vi "Connecting Points.vi"(1 "index":dbl[](array[numeric]), 2 "数组":dbl[][](array[numeric])) -> (0 "输出数组":T1(array[cluster]))   [LabVIEW 2016]
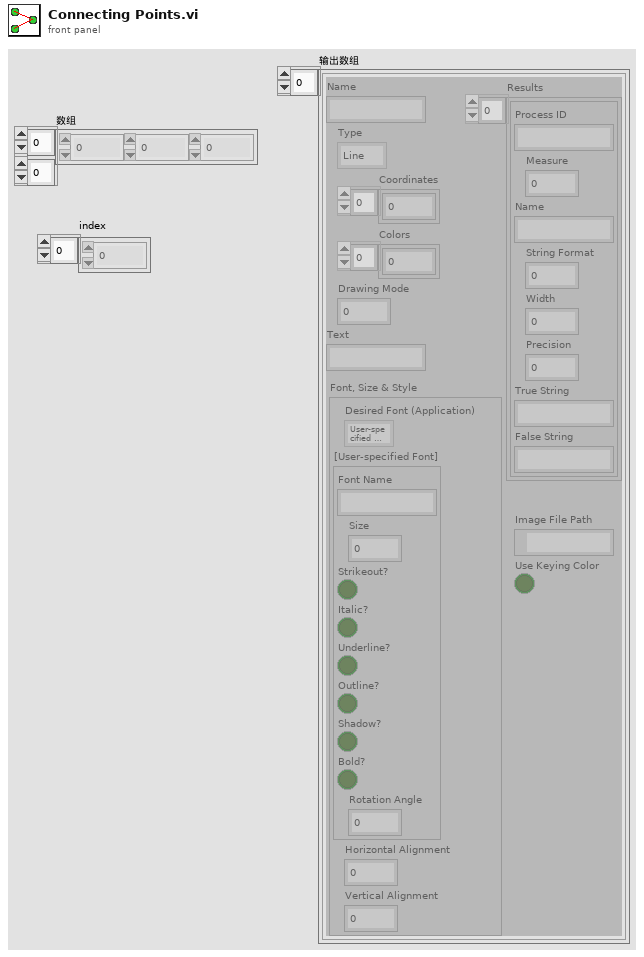
[diagram p1: front panel]
types:
  T1 = cluster{"Name":string, "Type":enum16{"Line", "Broken Line", "Free Hand Line", "Rotated Rectangle", "Oval", "Polygon", "Free Hand", "Bitmap", "Text"}, "Coordinates":i32[], "Colors":u32[], "Drawing Mode":u32, "Text":string, "Results":cluster{"Process ID":string, "Measure":u16, "Name":string, "String Format":u16, "Width":i16, "Precision":i16, "True String":string, "False String":string}[], "Font, Size & Style":cluster{"Desired Font (Application)":enum16{"User-specified Font", "Application Font", "System Font", "Dialog Font"}, "[User-specified Font]":cluster{"Font Name":string, "Size":i16, "Strikeout?":bool, "Italic?":bool, "Underline?":bool, "Outline?":bool, "Shadow?":bool, "Bold?":bool, "Rotation Angle":dbl}, "Horizontal Alignment":i16, "Vertical Alignment":i16}, "Image File Path":path, "Use Keying Color":bool}[]
  T2 = enum16{"Line", "Broken Line", "Free Hand Line", "Rotated Rectangle", "Oval", "Polygon", "Free Hand", "Bitmap", "Text"}
  T3 = cluster{"Name":string, "Type":enum16{"Line", "Broken Line", "Free Hand Line", "Rotated Rectangle", "Oval", "Polygon", "Free Hand", "Bitmap", "Text"}, "Coordinates":i32[], "Colors":u32[], "Drawing Mode":u32, "Text":string, "Results":cluster{"Process ID":string, "Measure":u16, "Name":string, "String Format":u16, "Width":i16, "Precision":i16, "True String":string, "False String":string}[], "Font, Size & Style":cluster{"Desired Font (Application)":enum16{"User-specified Font", "Application Font", "System Font", "Dialog Font"}, "[User-specified Font]":cluster{"Font Name":string, "Size":i16, "Strikeout?":bool, "Italic?":bool, "Underline?":bool, "Outline?":bool, "Shadow?":bool, "Bold?":bool, "Rotation Angle":dbl}, "Horizontal Alignment":i16, "Vertical Alignment":i16}, "Image File Path":path, "Use Keying Color":bool}
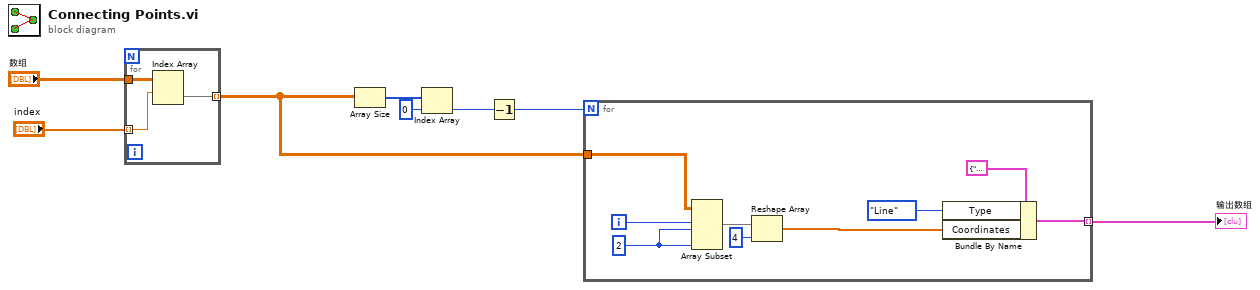
[diagram p0: block diagram]
diagram:
  n1 = for {
    tunnel: "数组" -> [w11]
    tunnel: [w10] -> w2 mode=indexing
    tunnel: "index" -> [w9] mode=indexing
    n2 = Index Array(array=w11, index (row)=w9) -> (element=w10:dbl[])  [unwired: 1 in]
  }
  n3 = Array Size(array=w2) -> (size(s)=w7:i32[])
  n4 = Index Array(array=w7, index=0 ("索引")) -> (element=w5:i32)
  n5 = Decrement(x=w5) -> (x-1=w4:i32)
  n6 = for {
    N: w4 -> [_]
    tunnel: [w20] -> w6 mode=indexing
    tunnel: w2 -> [w17]
    i -> [w16]
    w15 = 2 ("长度")
    n7 = Array Subset(array=w17, index (row)=w16, length (row)=w15, length (col)=w15) -> (w14:dbl[][])  [unwired: 1 in]
    n8 = Reshape Array(w14, 4 ("维数大小")) -> (w13:dbl[])
    n9 = Bundle By Name(cluster=T3 {"Name"="Line 1", "Type"=enum."Line", "Coordinates"=[606, 1151, 1346, 834], "Colors"=[16711680], "Drawing Mode"=0, "Text"="Your Text", "Results"=[], "Font, Size & Style"={"Desired Font (Application)"=enum."System Font", "[User-specified Font]"={"Font Name"="Tahoma", "Size"=13, "Strikeout?"=FALSE, "Italic?"=FALSE, "Underline?"=FALSE, "Outline?"=FALSE, "Shadow?"=FALSE, "Bold?"=FALSE, "Rotation Angle"=0.0}, "Horizontal Alignment"=0, "Vertical Alignment"=0}, "Image File Path"=path "", "Use Keying Color"=FALSE} ("Overlay"), "Type"=T2."Line", "Coordinates"=w13) -> (w20:T3)
  }
  "输出数组" <- w6
